vi "Parse.vi"(8 "Error In":errorcluster, 11 "object in":refnum<class "2021_25.lvclass">) -> (0 "Error Out":errorcluster, 3 "object out":refnum<class "2021_25.lvclass">)   [LabVIEW 2020, in "2021_25.lvclass"]
uses:
  2021_25.lvclass
  2021_25.lvclass/2021_25.ctl
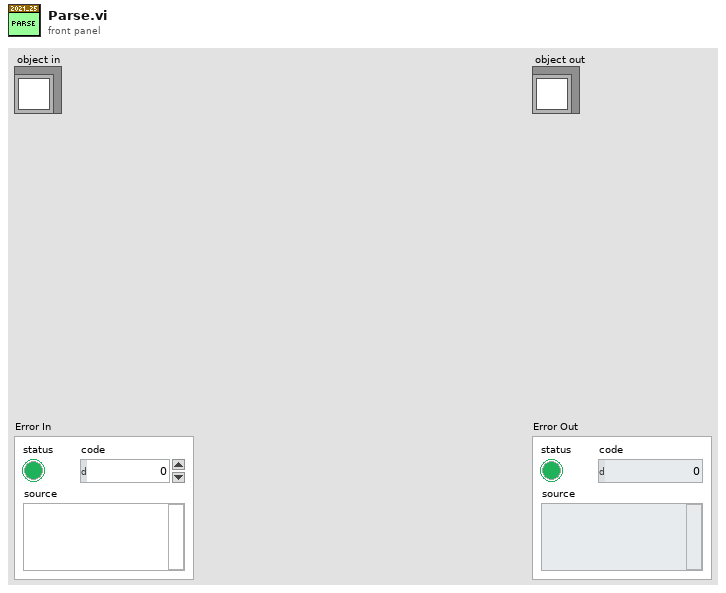
[diagram p1: front panel]
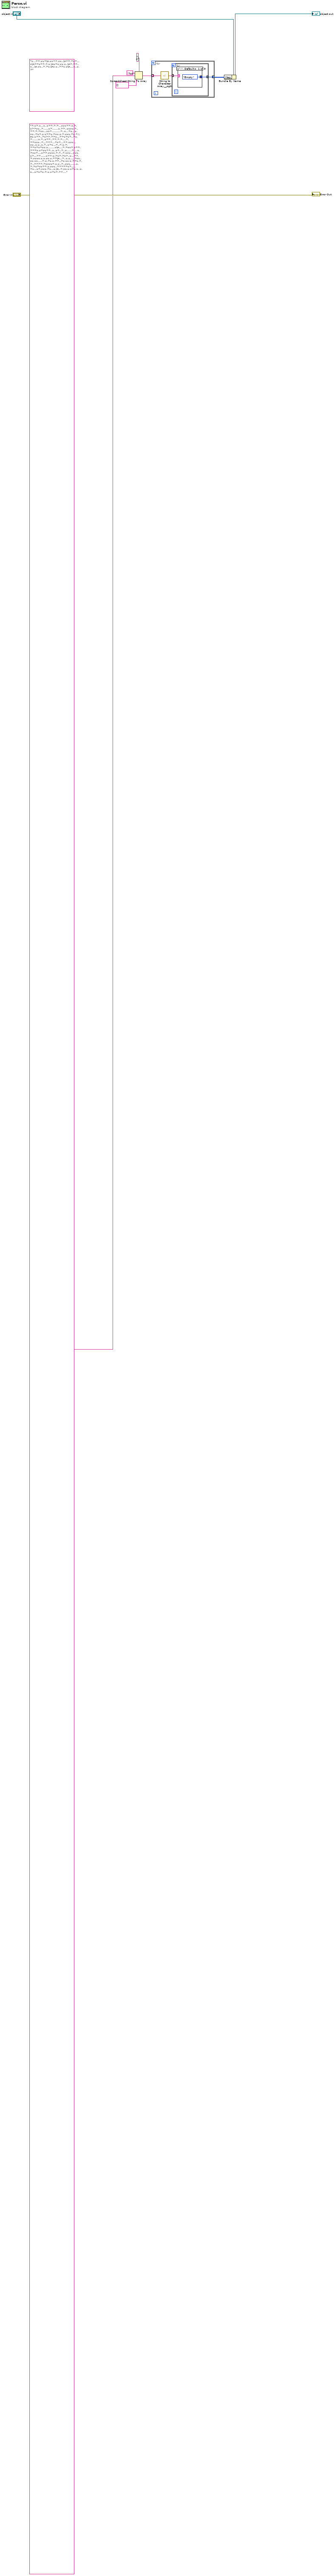
[diagram p0: block diagram]
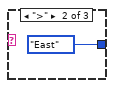
[diagram p2: hidden frame]
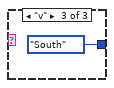
[diagram p3: hidden frame]
diagram:
  (unwired) "v...>>.vv>\n.vv>>.vv..\n>>.>v>...v\n>>v>>.>.v.\nv>v.vv.v..\n>.>>..v...\n.vv..>.>v.\nv.v..>>v.v\n....v..v.>" ("PuzzleInput")
  n1 = Spreadsheet String To Array(delimiter (Tab)="\n", format string="%s", spreadsheet string=">.v>.v...v..v>>.>.>...vvv>>.v.>.v>>vv..>......v>.......v.>>..vvvv.>..>>.>.>vv...vv>..........>..v...>v...v.vv..>v>.v.v>>v.>vv.v.>.vvv.>v.>.\nv.v>>..>v>>.>>v...>>v>v>..>v.>.......v.>..v>>..>>.>.>....>.>>vvv..>...>>>...>v>...>>.vvv...vv..v.v..v.>..v>v...>..>.v.>.>>v>v>vv.v........v\n....>.>vv>.v>>.>>>v.v>vv>>..v..v>..>..v......>....v.>vv>....v>>.vvvv.>.>..>.vvv...vvv.v>...>>......v>>.v.>v>.>v>..v...>>.>.vvvv.v.v.vv.v.>>\n...>..v.v.....>vv..vv.vv.....>.v.>v.v.>>..>v.vv.v.>>v.>.>..>>>>.>vvvv>.v.v..>..vvv.......v.>.>v>vv>>.v.vvv..>>>>>v>.....>v...v>.vvv.>v...v.\n..>.vv.v.v>v.v..v.v...v>v>v.>.v.v>v>.>>..>>v.>..>.>.......v>v..>...>.>.v..>v..v>vv>..>>>....vv.v....>.>..v.v..vv.>.>.v>>v..>>......vv.>.>v>\n.>.>.>.>>>>v..>.>.v>vvv.>v>..>v>vv.>v>.v...vv.>...>.v>.>>v.>v.>>.v>.>..v..>v>>...>.>.v>..>.v>>vvv.v.v>v>.>..vv....>.vv..>>v.v..vv..v.>.v>..\n>..>.>v>>v>>>>....v....>vv......v>.v.vvvvv.>..>v...>>v....>>v>>>>>.>>.......v..v>...>.>.v.v.vv....>>>v.>..v.>vv>...>v.>v>v.v..>.vv.>..>..>.\nv.v>>>.vv..v.v.>v>v>>>......v>.v.>v..>..>>>.v..v>.>..v...v.vv.....v.v>>.v..>..>.....v>....>>v.vv>.......>.>v....>>......v>.>.>.v.>.>>..v...\n>.v>..>>>..>..vv.vv>.>.>.>>vv.>v>>v.v>..>...v.>..>..........v..v.vv.>..>..>.v..v...vv..v>>>.>v....>..>>....>>>..v.>....>..v..>...>>.v.>>.>v\n>.>..v.vvv..vvv>.v..>v>>v>>.>.>..vv..vv>>v....>.v.>vv>...>..v....v..v..v..>v>.....>>vv.v.v>.>>...v.>..>vv....>.v.v.>>...>..>>.>>>>>>>.v>>v.\nv.v>>..vv>.v.v........>.v.v....>.v.vvv.>v>..>....vv.v.vv>.>v>v....vv.>v.v..>v.v>>...>>vv..>.v.>v.>v....v...v>vv>.>.v..>.v.....vvv>>..>...>.\n.v>v.v>..>v....v.>v>...vv>v..vv.v.>>...v....v>>.v>v>>>.vv>>.vvv..v...v>....v..>..>vv>>v..v.v.>>>>>.vv..vv...>..vvvvv.v.v>v>>..>v.v.v>..>>v.\n..v.vv>..v.v.>>..>v>.....>>.>v..>.>v.v.>vv>>>vv.>.v.>v>vv>>v...v>vv>>.>v>v..>.v>v>>..v>..v..v>v.vv.v>>.>v>>..>>vv.v>..v>v>>.v.v..>.>.v..vv.\n>>.vv>....>v.>v.>..>....v.>..v>>..>....vv..>.v>.>>..>.v....v.>v>v....v.>>.v..vv.vv.>..vv>.vv.vv>v.v>v.>..v..>.v>v...v...vvv>....vv>..v>.>..\n.v.v>>>v.....v...v..v...v.>.v...>>.vv.>>..v>..>v.v..v..v.v>.>>...>>....>..v>.>v.v.v..v.>>vv..v.>...>>vvv>v.vv.v.v..v.>.v.v>...>>......v..>>\nv.>..vvv.v>>v.v>>...v..vv.v.>.>v..v..>v.>v.>>v..v..>..v..>..>v>v.....v.v>.>v.v.>>>.vv.v.>>..>..v..>v>>....v.vv>>v>>v>v.>v..>>>v>..v.vvv.>..\n...>..>>.v....v>>..>.>v...v>>>..>....vv.v.>>...>...vv.vvv.v...>..v..>..v>.v>v.vvv>>v.>.vv...vvv>.>vv.>.v.vv...>.vv.>>>>>......>v>v..v......\n>...>...v.vv.>v.>>>v>>..v.v.v>>..>>>..>v.>>.>v.v.>v.>.......>.>>>...v..>>..>..>.>>.v.v>>vv.v>.v.....>>...>....>>......v>......>v>.>...>>.v.\n...v>v>..>...v>v.>>>vvv.v..v.vv>.v>..v>.v.v..vv.>v>.v.vv.>...>v..>...v...>v.v..v....>v>>..v...>..>...>...>>.v.v>.>..>.vvvv..>>>v.vv.>v.v>v.\n.>...>>....v...>>v>v>v.v......v.vv...>.vv.v.>..vv>.v..>..>.....vvv.v..v.>...vv.>>>vvvv.>v>vvv...v>.v.>v.>.v>>.v.v>vv.>..vv>.v>v>>>v.v...>v>\n..v..>v>.v..v..v>v.>v.v.>v>...>>v..v......v.>>>>.v.>.v.>v>v..>>>vv..>...>.....vvvv..>..>.>>>...>>>v>v..>...v.>....>.>...>.>v...>..........>\n>.....v.>..>.>>......>vv..v>...v...>>..>.v>>v....v>>...v>......v..v...>...>.>v.>.vv.>....>...v..>>>..>.>...v...vv.v..vv..>...>....>.......>\nv.>...>v....>..>>v.vv>.>>>..>vv..v..>>....vv...v..v.v..v>..>>>.>.v.>.v.v>..vv..>>.v.......v>.v.vv..>>v>>.....vv.>>..v>.>>v>...>vv>v>>v..>>v\nv>.v>.vv>>.>..v..>....v...v...vv>......v.v>v.>...v.vv>..>v.v>v>.v.>>..>>.>.vv>v.v.>.....>.v.>..v>.....vv.>>..vvv..vv.v..v>...>..>..>vv.>..v\nv>.....>v>>.>vv.vv.>>v..vv.>vv>v.vvv..v.v.>...v..>>v>.>vvvv.v...v.>.vvvv.>.v.v...v.>....>vv>..v..v..>....v.>.....vv.>.v.>.>.vv>vv..vv>v>>>.\n>vv..vv.>>.vv....v>>vv.v....v>>v.>>.>...vvvv..>.>v..v.v.v.......v.....>>>v..>.v>v>>v.>....vv>>.>v....vvvv.>>...>.v.v>...>>..vv>....v..>>v..\n....>...v>vvvv...v...>v.v...v.v...v>v>...vv....>>..vv.>....>>.vv.>.v>.>>v..vv>.v.>.>.>>.>.....v...v...v..v...>.vv.v....>.>v>.>.vv>>.vv.>>..\n.vv>.>...v>...>v>.vv>.....>.....v.>.>.>.>.vv...>v.>.v>.vv.v.>....v..v.>.v>.>v>v...v>.v..v.v....>.v.....vv..>vv.vv.>..>>...>.>..>.....>..v..\nv..v..>.vvv>.v.>vv.....>v.v...v.>.v.v>v.vvv.....v.>.....vv>...>>...v>>.>>..vvv>..v>>..>.>v>.v>v..v.>...>>v>v>.v.v..v..>v..>>.>..>.....v...>\nv.v.v..>>>....>.>>>v>>.v...>...v.>.vv>>..v.>..>>>...v..>v>..>>.>..v....>vvv...v>v>>>..>..>v>.>>>..vvvvvv.>vv.v...>.>v..v.>v....v.>..>.v....\n>>>>..v>v.....>.....>.v..v...>>....>...v..v...v>v.v>>....v...v>.vv>..>vvv.v..>vv.v...>......>v>>v..>...>....>........vvv>>.vv..>>.v..>>v.v>\n>v...>v>>>...v>.......v>v.vv...v.vv..>v.>.>vv>>vv...>vvv>...>.v>.>..>..>...vv.>>..v..>.v..v.v>v>>..>...v>v.>.>v....vvv...>v>...v.v..>..v.>v\n>.v.v..>..v.>.>.v.>..v..v.vv........>>vvv>.>v.v..>v.>..v.>..v>>....v..vvv>v..v>>>v>>...>.>>v>vv>....>v...>.>.vvv..>..v.vv.>....>..v..>.>>v.\n>...>v..v.......v..v..>v...vv.vv....v>vvv>...>>.....>>vv.v.v...>.>.vv>>>.>..>>>..>..>.>v.......>vvvv.>.>vv.v>..>v.>.v..>.v...v>v>.>.v>...>>\nvvv.>>.>v>....v>.>.>>v.vv...v.>>>>.vv>v>.>vv..v.>...v>>.v>..v.>v>..vv.>>vv.....v.>v>.>....v>....>vv.v.>v....v.v>>.>.v..v..v>.>>..>.....vv.v\n>>v.>>>...vv.vvv>>.>v>>v.>....v.>.>>v>..>.vvv..>v>.>.>>.vv..v.v>>v.>.v>v>>.v>.......>v>.>>>.....v...>...v>..>..v>vv..vv.>.v..>vv>..>vvv.v..\n>v...>v..v.v>>.....>....v>v..v>v.>..>.....>>..v>.>v.>.>.v>.>.v....>v...>.v.v.>vv.v.v.v..v>..v>v>..vv.v>...vv.v.vvvv>.>...>v...........>....\n.vv.>v.v.>>>>v..v.vvv>...v..>>.>v.>>v>>>.>v>.>.v.>...>..v>>>.....>v.v..v>.v..>.>.v>..v.v...v.>....v..vv.>>..>.vv>.v..v..>...>.>..>>vvv.v>>v\n.v.v>v.v.v.vvvv..>...v.vv.>vv..v>vv>>>..v>.v.vvvv..v>.>....>...>vvv>>>.v.>v>v.vv..vvv.v.v>.v.......>...>vv>v..>...>>...>.>v>>v..v.>....vvv>\nv>.v........vv>.v.....>.v...>.>..v>.........>.>.v>>....>>.>>..>..v.vv>>v...v..>v.v...v.v.vv.vv.....v>.v>>v.v>v>>>....>v>>>>v>v..v.>vv.vv.>.\n>vvv....>...vv.>>..v>>>.>>v....>...>.>vv..v>v.v.>>.v>.vv.>v>>.>v>....v.vv.v...v>.v.v>..>...>.>v>...v.....>v.>.v>....>.>.>.v.v>v.......vvvv.\nv..vvv...>>.v....vv.>.vv.v..v.vvv.>>>>..>>..>.....>v...vv.>.v.>vv...v>..>v...v....v>vv.>.>v..........>v...v>v..v>v..>.....v>.v>..>v......v>\nvv.>.>vv>v..>v>.vv...>.vv..>.v.>>>.>....v>v>>>>..v>....>vv..vv.>.v>.v.>...>.v.v>v>v>v.>..>v......v.vv>..>.>..>..>.v>vvvv.>...vv.>.>vvvv>>>>\n>..v...>v.vv.>>vv>>.>.>....v>...>v...>....>..v.....v.v.>>>>.>.>.>>.>.>..vv.>>vv..>...>>>.v....v.>>.vv..v>.>>>.>v..vv..>>>.>vv>>.....>vv.>..\n>.>>..vv>.>v.>>v...>..v>...>..>.>v>>v.v.....>.>..>.>v.v>.....vv>v>v..>v......>v..vv...>>>>>..v...>....>....>v.v>..>v.>.>.>.v.vvv..>>.v>v.>.\n>....v>>v>...>v.vv>>v..>>..v....>vv.v.v>.......>v.v.v.>>.v>vv>>..v..>...>.>......>>..>>.>....vv.>.v>>....v.>...vv.v>.>.vv.......vvvv......v\n.>..vv.....v....>>...v>.v.>>.vv..>.v...v.>>v>>>>vvvv....v....v.vv..v.vvv>>..>...>v.....>....>....v>v...>..>>..>..v.v.v...>>>.v.vv.v...v....\n..v.vv>.v>.v....>.v..>>>>v>.>vv>.....>v..>....v.>.v...>.v>>.>..v>v>...v>....>>.v..v...v.....>v.>...vv>>.>..v>.vv>v>v>...>>..vv.>..>.v.>.>..\n..>vv>.vv.v>v>v>.vv..>>>>..>>..>v>v>vv>.>.v>v.>>vv.>..>.vv.....>..>>.v.>..>.v.>.....v.v.vv.vvv..vv....>....v>.v...v>.>>v..v...vv.>...>.>.>.\n.>>>....>vvv......v>...>v.>vv.v.>>vv>.....v.v.....v.>.>.>..>>.>vvv..vv>.>>...v>..v>.>vv>>......>>.v>..vv..v..>v>v>.>.>.>>..v..v....vv.>.v.v\n.>.v..>.....v>v>>.>.>.>>>v>v..>....v....>>vvv.>>...vv>>v.v..v.>.>.>v.>..>>>v...>vv>.v>.vvvv..>.>.vv>.v..>.v..>..vv..>>>..v>>.>..>.vv>v.>v..\n..>v>>.v.>.v>>v>v..v.vvv.v..>>>v.vv.....v.v.>.vv>.>vv.v>.vvv..v.>.v.>v.vv..v>.>.v.vv>>...vv.>v.>.>.vv.>v.vvv....vv.....>...v>..v.>v.>v..vv.\n>.vv>.v>...v.vvv...vv.v>.vv>.v>vv>>v>>>>....>..v..v...v>v.>..v..vvvv>>v..v>v.v..>.>v...>...>v>>v.v.v>.....>v.v..>..vv>...>>.>...v.v..v.....\n..>vvv.v>.>>v...v.>>v.>vv..v...v.>.v>.>v.v...>>...>.>>.v....v>v....>.>.vv>>.v>v.v.v.v..v....v.>vv>...>..v>>....>v..v.>v.>>.>.>.>.v.vv..v.>v\n..>.......vv>v...>.>.>........v..>.>..v..v..v.>>.>>.v..v.>.>.>.v..>...>v.>v..>..>.v>>.v.v..>..vv.v>.>..v.>v>...>..vvv.v.v.vv.vv>>.v>>..>...\nv..>v....v.v>.>.>v..>v...>>.>.v>>>>v.v>>vvvvvvv.v.>vv.v...>v>.>..vv..v..v....v......>>v..v..>v...>.vvv.>...>v....>.v.v..>..>...v.>...v.vv>v\n>....v>.vv.....>>v.>>>>>.>.v..>.>v......>>>.>>...vvv......>.>>....v.>v.>..v>>>vv.>..>v>>....>.vv.>...v...v.v..>vv.>..v...v>.>v>.>>.>>.....>\n>.vv.v>.....v..>v...>..v....>>...v>......>>v>vv>...v.v....v>v.vv.v.v>...v...>....v....vv..v.>...>.>.>>>......vv...>v>vv.v...>v.v>..>..v...>\nvv>.v.....v>.vv>>..>..>.>....>>.>.>v...>>vvv...v..>>.v..v..>>v.v..v>>.>.v..vvvv.>vv>>.>....v.>..v>...v>v..>>v.vv>.>..vvv...>>.v...v..>..v..\n>>v....>>.....vvv...v>v.....v...>>>>...v>...>>>>v...v.v.v.>...>vv.........v..v>>v.v>v>.>>>>>.>vv...>..v.vv.v>..>.>.v.....>>v..>v>v.>v.>v>.v\n..>......v.....>vvv>....>>v>v....v>.>v.>v..>vv.vvv...vv..v.v.v.>...v.v>v.>>>....vv..>v...v.....vvv..v>.vv>v...v>.v.vvvv....>.>v.>v.>vv>vv..\n>v...v.>....>.>.v...>>v>..>..>..vv..>.>>vv.v>.>>..>.v.....>>.>>v.v.>vv>v>.....vv.>>v..v>...v>v...>...>.v>..>>v>.>>vv>v>.>.v.vv.>>>.>v.v..>>\n>.v>>.v.v>v>.>>..v>>.v>.v>v.v>....vv.vv..v..>...v.v>>..>vvvvv>.>.v..>>>..v..>>..v...v...>v.>.v.vv>.v>..>..>>.>.>.v.v..>v>.v.v>>v.vvv...>.v.\n....>.>...>vv.vv..v...v.>>>...>vvv>>.>.v.....vv>vv.>v.........v>v..v..vv.>..v>v.>v....v.>..>.....v..v>>>.....>.>>>vvv...vv>.v..v..vv>.>..vv\nv..vvv.>.>>....>v..v..v..v>>...v...v.>.v.>>.v..vv..>vvv..v....v...>.>>vvv>..>v.v.vv.vv.>.>.>vv..v>>>v.v.>......>.......v.v.v>.>v.....v.>v..\nv.vv.v.>>.>v.>vv>..>.v.>>v>.>v>.>.>v>.>.v>>.v..>........v.v..v..>>.v..>...v.v.>v>...>v.>.vv..>>.>v....v.>..v..v...vv..>>v..v>>vvv..v.v...>>\n>v..v>>v.>.>v..>v>..v...>...>v.v.>>..>v>.v>.>..v......v...v>>.>..v..v..v.>>....>>>>....>>....>.v>v.v>.v..>.>v>.>.v.v...v>...vv>>>..vvv>.v.>\n...>...vvv>>..>>.>vvv.....vv..v.v>.v..>>.v>>>vv>>v>>..v.>..>v>>v.>v.>.v>>vv>vvvv>.vv.>>.v....>..vv>....>>.>v>..v.>..v>......vv.v>v>.v>..>..\n.v>..v>>..v.vv.v..v>.>.v..v.v..vv.......>.>...>.>..>v.vvv...v..vvvvv.>>.v....v.>v.vvv>v>.>.>..v.vvv..>..>>v..>....>....>v.>...v...vv..>v>v.\nvv.v>...v>>.....>v>v...vv>.>.>>.vv..v...v.>.>..>.v.v>>.>..>v...>.v..>.v>.v...>...>.>vv..>vv....>.>.>.>>.>.>>>>.v..>.vv...>>v..>vvv..>.>v>..\n>..>v>.>v.>vv.>vv.v.v>.>.v..v..>v>>.>..>..>.v>.v.v.v>>..>....>>.>>>v.v....v.>>>...>v>v.>.>.v.vv.>>.vv>..>.v........>v>v.>..>.>.>>v.>..>.v>v\n..v>>>>v.>vvv>...v..>.......>.v.>vv>v....>.>>>..vv.>..>>v>>v>.v>...v.>...v.v>v.....>v>.vv.>>>v>..vv.....vvv..v.>.>.v..>.>.v.>..v>......>.>.\n>.v..>.>..v>vv.v..vv..vvv>>vvvv..>v>v>v>v...v.v>>>>v.>>v.>v..>vv..v...>v.>v..>vvv.vvv..v...vv...>.>>v.v.....v..v.>.vvvv>v..>v.>.v.......v..\nv.v.v.v.v>.>.>v.>.v>>vv.v.v>.>.v>>..v>>>....vv.>...>...v.vv>.>...v..vvvvvv.v..v.>.v>v>v..vvv........>..>>...>..vv>v.......v>>v..v....v>.v.v\nv..>>.>..>...>.v>vv...>......v>.>..>v....>v....vv..v.>>.>.>>.......>v..v.>>.v.v>..>.v..>v..>.>.vv>.vvvv>.v>.v>v.>>v.v>v>vvv...v....v>v>.>>.\n.>>.>v.v>..>.>v........v>.v.v.v>.........>v>.>>v..>vvvv.>v.>>..v...>.vv>..>....>.vv.vvv.>>>..>>.v>v.v>.>.v>....vv...>v>>.....v.>..v.>.>>>v.\n>v>>.v>.v>v...v..v..v>>...>.>>>..>..>...vv.>v>>>.v....>>.......v..v...>.v..v..v.>vvv.......>vv>v.....v..>>v..>.>vv>>..v>.v..>..>.v..v.vv>.>\nv...v>v.v.>>.vv.>>...>...vv>....v.v>..>>..>>>...>>.>..v>v.>v..>..>.v....>.>..>.....>.vvv.v..>...v..v>v..>.v....v>.vv>v.v>.v.>.....v....>..>\nv....v>.v..v>v>.v>vv.>.>v>.......>......v>.v.>..v.>...>...v...v.v.>...v>>v>.v.>v.>>...v>v.v.v>...v>v.vv.>v..>>>.>v>.>v.v.v...>.vv..>..>.vv.\nv....>.v>..v>.v>.>..>..>.>vvv>>.v...v..>vv..>......vv.v..>>...>>.>>..>v...vv..>.v>.>v>v.>.>>...>.v.v.>..v>>>..>.vvvv>..v.>...v.>.>..v>.v...\n>.vv>.v.>v....vv>.>>.v>>v....v.>v..v..>>>..vv..>.>>>.>>.>v.>>.v>>..>.>>...>.....>.>v..>.......v..vv..>>v.>>...vv>>.v.v>....v.v>>.>>..v>v.v.\n>v...>>.....v.vv..v>.vv..>.....>....v.v>..>>...>..v..>>.v>>.v>v.v.vv.v>....v....>>.v>....>>vv......>>.v>..>.vv.>..v.v>.v>.vv.>...>>.....>vv\nv>v...>.>.>....v.vvv.>vv>.>.>..>>v....>v.......v...>v.v.v...>v>.>.....>v....>.v..v.v.....>.vvvv.v.vv>.v>>...>...>..v>>>>...v>>.v..>v..v>...\n..>>v>>vv..>.>>.>...v>>>vvv>v..vv.>...vv..vvvvvv.>>..>v..>.>>>.v.v.vv..v.v.>.......v>.vv...v>.v......vv>v.>v.v>.>>>v...>>vv>.>.>....v..>v>>\n..>v.v..v>..v.>vv>vv..>.v.>v....>....v..v>>v>.>.vv....>v..v>..v..v>.v>.>>>>>.....>>.....>>>v.>>.v>..>>vv..>>>v.v.vv..>>..vv...>>.>>...>v...\n..>v....v.>v.v.v>.>>v.v>...>>v.v>...v.v...>vv.>>..>>......v.>>vv...>.>....>v>.v...v....>.>.vvv.>>>v..>>vv.vv..>v.....>>....v>>v>.....>....>\nv........>v..>.>vv....v.v>>.v>.>>v>.vv..>...>..>v.vvvv.v.>....>.v>>.>v>>>.v.>.>.....v.v>v.v>v.v.>v>..>v>>v..vv>>>..v..v>>.>v...v>...v..>>v.\n.>..>>.v.>v......>.vv>v>.v.>.v.v..>>..vv...v..v.>>.v>.v>.....v.>..>.v.>v>.>..>v.v...vvv..v..>.>.v>vv>.v>....v>.>v..v>v>>>.vv.....v...>v>>v.\n.....v>..v>>>v.v..>>vv.v..v>.>...v..>.v.>>>v.>.v>.v>v>.>>..v.....v..v>vv.>>...v.v.v.vvv>>>>..>vv..v>....>...>>.>....v>.>>..>>....vv>.vvvv.v\n.vvv..>.v>vv>>>.>.v>..>>.>..>.vv.>....>.v..v>vv...vvv..vvvv.>.v.v.>>vv>..>>........>>..v...>.vv...>v>.v.>v.v.>..>.v>>>>.....>.....v>.>..>.>\n.vv.>>vv.v...v.v...>v>>>>v..v...>>......vv.vv...>v..vvv.vv.v...v.v>....>v.v.v.>....>...v..>v...>v>....v...>....>.>>.>..>>v>.v>v....>..vv.v.\nv>.v.>v...vv.>.v.>.....>.v.vv.>>.>....>..v.v.v..v>v.v>vv.>>.>v>.>....v.>.>.>v..>.vv..vv....>.v.>..>vv.vv>>v>...>v>>>v>...>v.>v>.v>.v>.v>v..\n..>>>.vv.v..>.>..>....>...>>>.>..>>>v..>..v...v>v>.>.vv....v.v......v.>.>>>.v.v..vv.v..>.>..>>.>>...>.>>..v.vv..v>.>vv..v>.>vv.>..>.>..>...\n..>.>...vvv.v.v..>.v.>>v.>v>>....>..>.>.v>>vv>.>>.v...>...vv>>>vv.v...>.vv..v..vv>..>v..>.>.>.>.>v>>.>..vvv>.>v....>v....v>>>............v.\nv.vv.>..>vv...v.......>......>>>v.v>.....>.v>>.v.>..........>>.v.>.>..v>.v.v...>..v>.>>>>v>..v>v.>.>...>.>....vvv.....vv.v..>.......v>v>.>>\n.>.vvv.>.>vvv...>>.>v.v...vv.v.v>...v..v>>v.v..v.>>vvv...v>>>.v...>..>v..v>>v.>v.>.v.v..v>v.>...vvv..>v......vv>>>>.>>.....v.>>>v.vv.>..v.>\n.vv...>>>..vv..vvv....v>v.v>v>v.vv.>>vv.>vvv>..>...vvv...v.>.>...>...>........v.v>.v>>...v>...>>.>v.>...>.vvv>...v>..v...v.>v>>..>>..v.>v>.\n.....>>.v....v..v>vv.>..v...>vvv>..>....v>..>.>..>v.>v....v>v...v...v..>...>>v.>>.vv..v..>.v..>.v.v>v>vv.>.>vvvv...>.v.v.v....>>v..vv.>>.>.\n....v>.v>v>.>.>.v>.>...v>...v>>>...>>.>v>.....>>.>..vv..v..>>..>.>v.........>v....v..v.v>...>....>v.>v>>....v..v..>>v.>....>....>v.>..>.vv>\n.>>.v.>.v.v.v...>vvv>..v.v>v..>v..>v...>....vvvv.v>>v.>>v...>..v.vvv..>..>>v..v...>v>>vv.>>..vv..v..v>...v...v....v...v....>vv>>.vvvv>.v...\n..vv..vvvv.vv...>.v>>.>v>>>>>.v.>..>.>.v.vv>>.>>....vvv>.>>.v.>.v.vv>v>v.>....>v.......>.>.>.vv..v.v>v.v...>..v.>..v>...v>v>>>......v>..>v.\n>.>>.v.v.>v>v.v>.>vv..>>.vv.>>vv>....>.v.....v.>v..>>>.>.>..v>.>v...v...v.>..>.v>v>..vv>..v.....v.>.v>.>>....v...>.v.....v>vv.....>>>v.v>.v\n.v>.....v...>.>...v>v.v..v.>v.v.>>v>.vvv>.>.v.vv.>v>v>v>v>>.vv..>>v.vv>.v>>.>vv..v>..vv.vvv.vvvv>.>.v.>.>.>vv>.>...v>.v>v...vv>v..v>v..>...\n...>..v.......>v.v.v>v.....vvv...v..>>vvv>.>...>..>.v.v.>>.v.v.>.v..vvv..vv>v>v..>..v.>..>v.>.>...v>.vv.>>.>v.>..v>v>....>.>.vv..v>....vv..\n.vvvv.v.>.v..>.v.>v.v>>..vv...>>v.>>.>.>.>v.v.v.v>v....v..>v....>>.>v>v.....>.>..vv....>.vv...vvvv.vv.vv...vvv.>.v>v.>.v>..v.v>vv.>..>.....\n>..v.v..>.>>.v>..>...>.>>.>>.>..>.>....>v.v>.>.v.....v>.v>.vv.v>...vv.>.vvv>>v>.>.v..>.>.v>v>.>..v..>.>......>>.......vv.>..>.v>vvvv..>vv.>\nv....v.vv...>.v.v..>>.>....v>>........vv.>.>>...>.>...v..>.v>..>..>>v>....v.v..>..>v.vv.>.>>.v.>>.>vv>>.>v>.v>>>.v....>....>...v>>..v..v.v.\nv.v.v...>>v...>>>.v.vv.vv.vv>>>.v.>...>>v.......>v.>vvv.>>.vv.......vv...v>..v>.>>.v..v>...>.v..vv.v>..>v...v.vv>.>>.v..>.v.>.>..>>.vv>...>\nv..>vv.>v>.>v.>.>>>vvv>..v.>>>v>.>v....v.>v>.vvv>..v>....v..>>..v..vv.>...v.>.v......v.>.>.....vvv..>vv>.>...>.vv>....>>..v>..v.v..>>v..>v.\n.....v.>>vv.v>>.>vv>.>..>...v>>..v>....>.v.>.>...v>..vv>v>..>..>.>......vv>.>.vv>.....v>...vv..>..>v.v.>.>.vv>.vv.vv>.vv.v>>>..>....>.>.>v.\n.>v..v.vv..v.v.>v..>.v>>v>v.vvv>>...vvv.....vv..>.v>...>>>.v....v>>.>v>.v.vv>....>>>>..v.>.>.v.....v>>v..v....>..v....v>...>>v.>v>v...v.v..\n.>v.....v..>.v..>...v..v.>vv.vv.>.>v.>...>...v>...v.v.>..>v..>..>v.v..>.v.v>v.>.v..v......>...v.vvv.v>>v.>.v.vv..>>v..v>>.v.>>.v.v>>>....vv\n...vv.>v.>..v>>..v.>.>vv.vv...>.....>v>.....v..v..v.v.>>..vv.>v.>..v........v.v..>>v.>v.v..>...>v.v..vv>v.v.v>..v>.....v.v.>.v....>>>v>>..v\n...>v.v.>...vv>.v.v.....v..v....>>..v.>v>vv>>.......>v..v.vv..>.>>>vv>v>>>.v....vvvvv.v..v>.v.>v>v>>..v..vv..v.vv>>v..>.>..>....>..>.>>.v>.\n>>..>>...>..v>vv.>>>...vvvv....vv.v>.vv.>.v.vv>>..vv..>..>>>..>>..vv>>.>vv>>.>.>..>vv.>.>v..>>.>.v>....vv>v>..vvv.vv.>v.>v>>....vv.vvv...v>\n..>>v>..>>.v>vv>....>..>>.v>vvv.vv..>.v>v..v.>>.vvv>.>.>v...>v.vvv.>.v.>v>v.>..>.v>>.>.>v..v..>v>>v>.v.>.>.v.>...vv...v.......vv.....>.v.>.\n>..vv>>v...v>v.>vv>.v....v.vvv.>......>v.v>.vv>..>>>v....>>>.>...v>>>....>...v..>..v>vv..v>v...>vv>.v..v..v>.>.>.>..vv>>v..v>....>>..vv..>.\n.>.>v>vvv.v..v.>v.>...v>.>v..>vv.>..v.>v>.v...v>.>>vv..........v>.v.vvv.>>>..v>vv.>>>v>..v....v..>..v.>>..>.>.v>v.v>.v>.v...v.>>.v....vv...\n....>>.v..>.......>.v.v>>>vv>>..>v>v...>.v..v>.vv.v>>vvv....>vv>v>..vvv.>>>.v..>>.v.>.....>vv>>....v>vv>v..>.>...>.>>v......>..>v..v....vv.\n.vv..>.>..>..v>...>v.vv.>..>v.>..v>v..vv>>>..vv..>vvv.....>...vv>.........v..>..v..>>.>>v.v...>>v>v>..v>>.v>.v..>v.vv>vvv>>>..v>.vv..>>.v.>\n.>vv.v.v..>.>...>..>v>..>...v.>...>vvv.>....v...>..vv...v>...>vv>v.v..>v..>v.>...v.v>v.>.v>v>>>v>..vv..v.>>v>.v>..v...>v>>..>.v.v.>>..>.v.v\n...v>..v.v..v>vv.....>..>..>>......v.v.>v.....>v.v...vv.v.>v>>>.....vv.>>v>>......v..v>v..vv>>v....v..>..>v>>>.v..>.>...v...vv>vv>v...>.v>.\nv.>>v.vvv.vv.vv.>.>.v.v>v.v>..v>v.>>>..>v>.v....>v....>>.>>..v.vv...v.v....>.>..>........vv.v.>..>>.v.v>...v>v...vv.v>>.>v>>.>>vv>.v..>v>vv\nv.>v.>v>.vvv.>v..>..>>>...v.>.v...v.>>.>..>>.v.>v..>.vv.>....>>vv>....>..>>vv>>....>v>.v..>.v>.>...v..v..>v>>>..v...>...>.>v>.>v.>.>.>.>.vv\nvvv.>>v>>v>.>..v>v>..v>v.>>v.v...v..v.>vv...vv.>.v>>>vv>.v.>v..v>>.>>vv..v....>.>v.>>v.>.>....>>.>.v.vv>.vvv..v...>..vv..v......>vv.>>>v>..\n.>.>.vvv....>v>>.>.v.vv.v>>.>>...>v>..v.>v.>>>>v.v>v.>v...>>>>>...v....>..>v.>>>.......>...>v.>vv.>.v.vv..>>......v.>..>...>.>v.>v>..v.vv>.\n..v>..>vv.>v>>..v.>.v....v>.v>>v.v...>vv....v..>.>....>.>v.v.v.v>..>.>.>.v.>>.v..v.>>v.vv>>>v>.v..v...v.v>vv>>vvvv>.>...>v.v.v..>>>.v>>.v.v\n.>...v>v>>..v.>>.>v.vv>.vvv>.v....v>..v.>.vv..>.>>.>.>v>...v.>v>..vv>.vvvv>.>....>..vv>.v.v..>v..v>...>...vvv.v>>>>>>..>.>.>...>..vv.>.v..v\nv...>..>.>vv..>.>v..v.>>.v>>>.v>>...>.....vvv.v.>v..>..v..v...vvv.vv>..v>.>.vv>v...vv>>>v...v.>v....v.v..>..>vv.>v>vv.vv>>>..>v.>vvv.>v.>..\n>v...v...>>.v.>.>>.v>>.vvv>>v>vv..>>..v>>.>..>.>v>>>v...v..>.>v..>....vv..>>.>>......>v>>>..v..v..>>>.>....>......v..>>v>>.>>...vv.v.>vv>v.\n>.....v.....>v>.>.....>v.v.>.v>vv..>.>>....vv>..>v..v>.v...>.v.>v>v.>vvv..v>>v..>..v>>.>...>.>>.>..>.vv>>.vv..>>v>>.>.v.v.v.>vvv>v>>v>vv.v>\nv.>..>v.v>v.......>v......v...v>.vv..v>...>.>.....v.>..>.>....>...v.v>v.v.....>....vvv>..>v.v.>vvv.v.v.v>>>..>v>.>.v>..v.v>.>vv.>.>.v.vvv.v\nv...>.vv>.v..>.v>.....>>vv>.v..>>>v.>>..>.....>v...>>..v.>.vv.>..>..>v.>>>>>vvv....vv.>v..v>..>.v>..v.>...>v..v.>..>v.>.vv.>vv....>>v.vvv>.\n>..>>...>.>.vv>..>v>..v..v>.v.>.>vv.>v>.>>..vv.>..vv.v>vv>v>.vv..>>>..>v...>.>v>v>>>.........>>>...vv.>.....v.vv>.>.vv>.....v.v..>...v.vv..\nv..>>..vv..v..>...>>.>>>..>..>.>v..>..>.>.vv.>>...>.>.>v>.>..>>.vv.>..>.vvv>>....>>>>....>v.>>>>.>>..v.v.>vv..>..v..>.vv>v....>vvvvv>v....>\nv...v.>v>.v...>>v.>.v>>.v.v...v.>..>..>>>...v.......v>>>>>.>.v.v..>...v.>v>v.v....v....vv>vv.>.>v>vv...v..vv.v.>>v..>.v.v.v...vv..v.>v>.>v.\n.>v>.vv.v.>.>.>>v.>>...v.vvv.v>...>>.>>.>.v...v....>..vvv.>....v.vv.>..v...>>..>...vv.>.>v>v..>>>.v.....>.....vv.v..>.>>>v.vv>vv.>......>.>" ("PuzzleInput"), array type (2D Dbl)=string[] []) -> (array=w3:string[])
  n2 = for {
    tunnel: w3 -> [w12] mode=indexing
    tunnel: [w10] -> w2 mode=indexing
    n3 = call <userlib>:"String to Character Array__ogtk.vi"("Input String"=w12) -> ("Character Array"=w11:string[])
    n4 = for {
      tunnel: w11 -> [w14] mode=indexing
      tunnel: [w13] -> w10 mode=indexing
      n5 = case shown="\".\", Default" w14 {
        tunnel: [enum16{"Empty", "East", "South"}."Empty" enum16{"Empty", "East", "South"}."East" enum16{"Empty", "East", "South"}."South"] -> w13
        frame ".", Default {
        }
        frame ">" {
        }
        frame "v" {
        }
      }
    }
  }
  n6 = Bundle By Name(cluster="object in", "Map"=w2) -> (→"object out":refnum<class "2021_25.lvclass">)
  "Error Out" <- "Error In"
